vi "Test_WriteValue_CheckDisk_ValuePresent.vi"(8 "error in (no error)":errorcluster, 11 "TestCase in":refnum<class "TestPersistToDiskTransport.lvclass">) -> (0 "error out":errorcluster, 3 "TestCase out":refnum<class "TestPersistToDiskTransport.lvclass">)   [LabVIEW 2017, in "TestPersistToDiskTransport.lvclass"]
uses:
  TestPersistToDiskTransport.lvclass
  TestPersistToDiskTransport.lvclass/TestPersistToDiskTransport.ctl
  Source/Concrete/PersistToDiskTransport/PersistToDiskTransport.lvclass/PersistToDiskTransport.ctl
  <vilib>/Utility/error.llb/Clear Errors.vi
  Source/Concrete/PersistToDiskTransport/Format Persistent Filename.vi
  Source/Concrete/PersistToDiskTransport/PersistToDiskTransport.lvclass
  C:/Git/composed-transport/Source/ITransport/ITransport.lvclass
  externals/variant-extensions/Source/Format Type String.vi
  Source/ITransport/ITransport.lvclass
panel:
  out "Test File Path":path
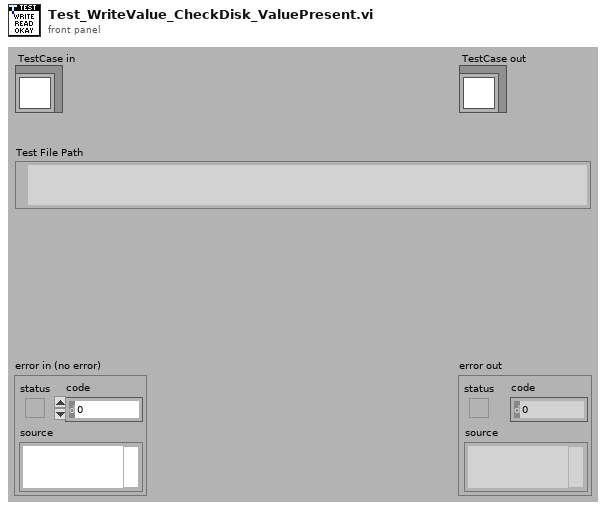
[diagram p1: front panel]
types:
  T1 = typedef "PersistToDiskTransport.lvclass/Recovered Value.ctl" = cluster{"Datum Name":string, "Datum Value":variant, "Last Publication Time":timestamp}
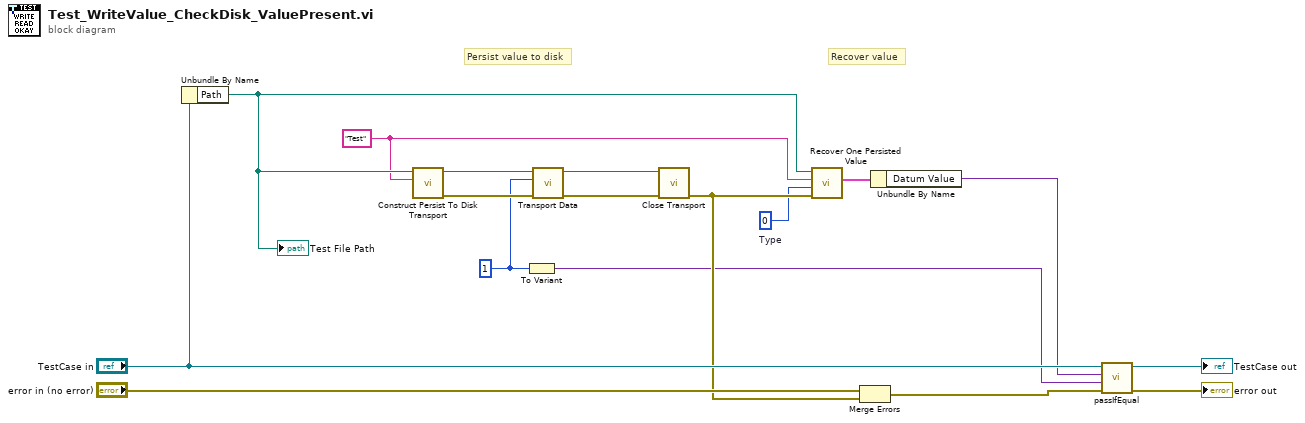
[diagram p0: block diagram]
diagram:
  w7 = 0  # Type
  w1 = "Test" ("Key Name")
  w4 = 1 ("Test Value")
  # "Recover value"
  # "Persist value to disk"
  n1 = Unbundle By Name("TestCase in") -> ("Path"=w2:path)
  "Test File Path" <- w2
  n2 = call "Construct Persist To Disk Transport.vi"("Datum Name"=w1, "Folder Path"=w2) -> ("error out"=w16:errorcluster, "PersistToDiskTransport"=w11:refnum<class "PersistToDiskTransport.lvclass">)  [unwired: 8 in]
  n3 = To Variant(anything=w4) -> (Variant=w3:variant)
  n4 = call "Transport Data.vi"("error in (no error)"=w16, "Value"=w4, "ITransport in"=w11) -> ("error out"=w10:errorcluster, "ITransport out"=w17:refnum<class "PersistToDiskTransport.lvclass">)  [unwired: 7 in]
  n5 = call-dynamic "Close Transport.vi"("error in (no error)"=w10, "ITransport in"=w17) -> ("error out"=w8:errorcluster)  [unwired: 9 in]
  n6 = call "Recover One Persisted Value.vi"("error in (no error)"=w8, "Data Type"=w7, "Datum Name"=w1, "Folder Path"=w2) -> ("Recovered Value"=w6:T1)  [unwired: 6 in, 1 out]
  n7 = Merge Errors("error in (no error)", w8) -> (w12:errorcluster)
  n8 = Unbundle By Name(w6) -> ("Datum Value"=w5:variant)
  n9 = call-dynamic "passIfEqual.vi"("error in (no error)"=w12, "y"=w3, "x"=w5, "TestCase in"="TestCase in") -> ("error out"=→"error out":errorcluster, "TestCase out"=→"TestCase out":refnum<class "TestPersistToDiskTransport.lvclass">)  [unwired: 6 in]
